vi "FindRow.vi"(2 "# Rows":i8=4, 3 "Image In":T1 {"Dialogs" format="%.0b"}) -> (0 "Row":i32, 1 "Image Out":T1 {"Dialogs" format="%.0b"})   [LabVIEW 2024]
doc: "This VI takes a binary image and a number of rows as inputs (i.e. the number of regions into which the user wishes to divide the image. It will return an integer value equal to the row that has the highest percentage of pixels. For example, if used with a binary image produced by a red mask, this vi will tell you in which region of the image the largest red object exists. If used with a motion mask, this vi will tell you in which region of the image the greatest motion exists."
uses:
  <userlib>/ImageProcessing/QTLIB_2595_LV86/QT_Image.ctl
panel:
  out "Relative Percentages":dbl[](array[numeric])
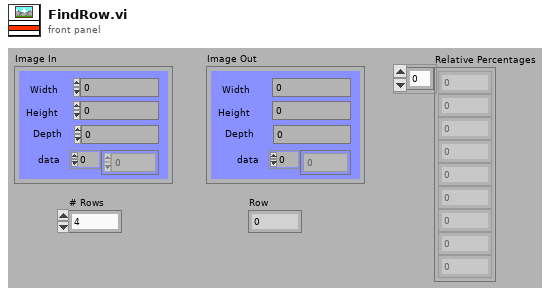
[diagram p1: front panel]
types:
  T1 = typedef "QT_Image.ctl" = cluster{"Width":i32, "Height":i32, "Depth":i32, "data":u8[], "Compressed data":u8[], "Color table":u32[], "Duration":i32, "Options":i32, "Timestamp":i32, "ID":i32, "Reserved":i32, "Dialogs":u32}
  T2 = cluster{"left":i32, "top":i32, "right":i32, "bottom":i32}
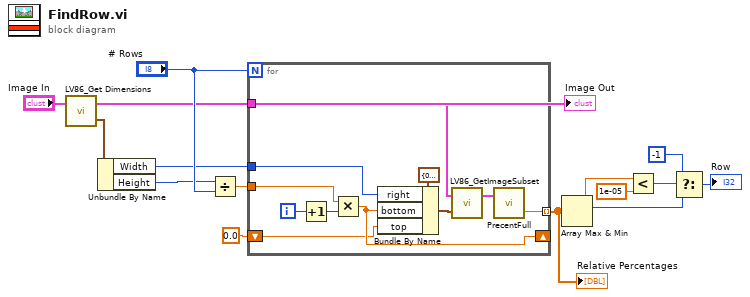
[diagram p0: block diagram]
diagram:
  n1 = call <userlib>:"LV86_Get Dimensions.vi"("Image In"="Image In") -> ("Dimensions"=w8:cluster{"Width":i32, "Height":i32}, "Image Out"=w1:T1)  [unwired: 1 in]
  "Image Out" <- w1
  n2 = Unbundle By Name(w8) -> ("Width"=w11:i32, "Height"=w9:i32)
  n3 = Divide(x=w9, y="# Rows") -> (x/y=w14:dbl)
  n4 = for {
    N: "# Rows" -> [_]
    tunnel: w1 -> [w26]
    tunnel: w11 -> [w21]
    tunnel: [w20] -> w12 mode=indexing
    tunnel: w14 -> [w19]
    shift-right: [w18] -> _
    shift-left: 0.0 -> [w17]
    i -> [w22]
    n5 = Increment(x=w22) -> (x+1=w16:i32)
    n6 = Multiply(x=w19, y=w16) -> (x*y=w18:dbl)
    n7 = Bundle By Name(cluster=T2 {"left"=0, "top"=0, "right"=0, "bottom"=0} ("ROI"), "right"=w21, "bottom"=w18, "top"=w17) -> (w23:T2)
    n8 = call <userlib>:"LV86_GetImageSubset.vi"("ROI"=w23, "Image In"=w26) -> ("Image out"=w25:T1)  [unwired: 1 in]
    n9 = call <userlib>:"PrecentFull.vi"("Image In"=w25) -> ("% solid"=w20:dbl)  [unwired: 1 in, 1 out]
  }
  "Relative Percentages" <- w12
  n10 = Array Max & Min(array=w12) -> (max value=w7:dbl, max index (indices)=w2:i32)  [unwired: 2 out]
  n11 = Less?(x=w7, y=1e-05) -> (x < y?=w5:bool)
  n12 = Select(t=-1 ("f"), s=w5, f=w2) -> (s? t:f=→"Row":i32)
